vi "kForce2RST.vi"(9 "Encoder Count Sync":i32, 11 "Force":dbl) -> (1 "Saturation Count":u16, 3 "RST Array":i16[](array[numeric]))   [LabVIEW 2010, in "KevLib01.lvlib"]
uses:
  KevLib01.lvlib
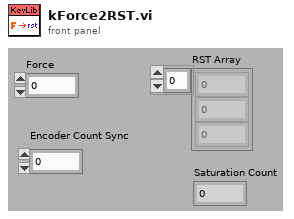
[diagram p1: front panel]
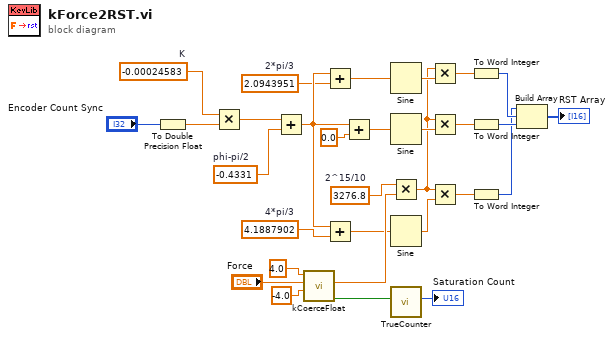
[diagram p0: block diagram]
diagram:
  w30 = -0.4331  # phi-pi/2
  w28 = -0.00024583  # K
  w1 = 4.1887902  # 4*pi/3
  w8 = 2.0943951  # 2*pi/3
  w17 = 3276.8  # 2^15/10
  n1 = To Double Precision Float(number="Encoder Count Sync") -> (double precision float=w27:dbl)
  n2 = Multiply(x=w28, y=w27) -> (x*y=w29:dbl)
  n3 = Add(x=w29, y=w30) -> (x+y=w10:dbl)
  n4 = call "kCoerceFloat.vi"("lower"=-4.0 ("lower limit"), "input"="Force", "upper"=4.0 ("upper limit")) -> ("coerced?"=w13:bool, "output"=w11:dbl)  [unwired: 7 out]
  n5 = Add(x=w10, y=w8) -> (x+y=w5:dbl)
  n6 = Add(x=w10, y=w1) -> (x+y=w2:dbl)
  n7 = Add(x=w10, y=0.0) -> (x+y=w6:dbl)
  n8 = Sine(x=w5) -> (sin(x)=w23:dbl)
  n9 = Sine(x=w6) -> (sin(x)=w22:dbl)
  n10 = Multiply(x=w17, y=w11) -> (x*y=w18:dbl)
  n11 = Sine(x=w2) -> (sin(x)=w24:dbl)
  n12 = call "TrueCounter.vi"("True?"=w13) -> ("True Count"=→"Saturation Count":u16)  [unwired: 10 out]
  n13 = Multiply(x=w18, y=w23) -> (x*y=w4:dbl)
  n14 = Multiply(x=w18, y=w22) -> (x*y=w7:dbl)
  n15 = Multiply(x=w18, y=w24) -> (x*y=w3:dbl)
  n16 = To Word Integer(number=w4) -> (16bit integer=w20:i16)
  n17 = To Word Integer(number=w7) -> (16bit integer=w21:i16)
  n18 = To Word Integer(number=w3) -> (16bit integer=w19:i16)
  n19 = Build Array(w19, w20, w21) -> (→"RST Array":i16[])
